vi "sätt_ström_supersub.vi"(5 "Spänningsaggregat":refnum<visa-resource-name>="COM4", 7 "Strömmultimeter":refnum<visa-resource-name>, 8 "error in":errorcluster, 9 "voltage_max":dbl, 10 "current_in":dbl) -> (0 "error out":errorcluster, 2 "current_act":dbl)   [LabVIEW 2024]
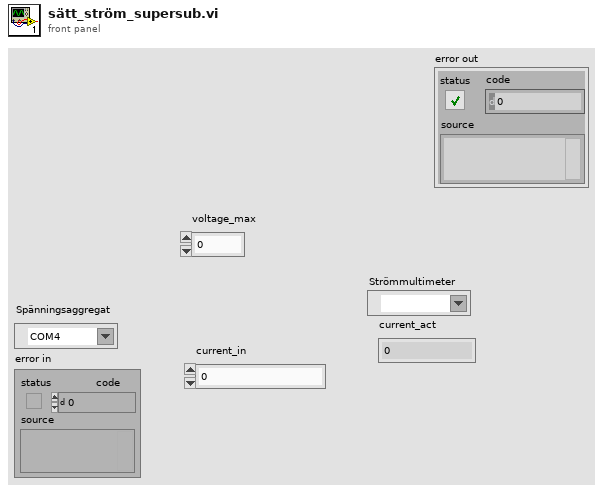
[diagram p1: front panel]
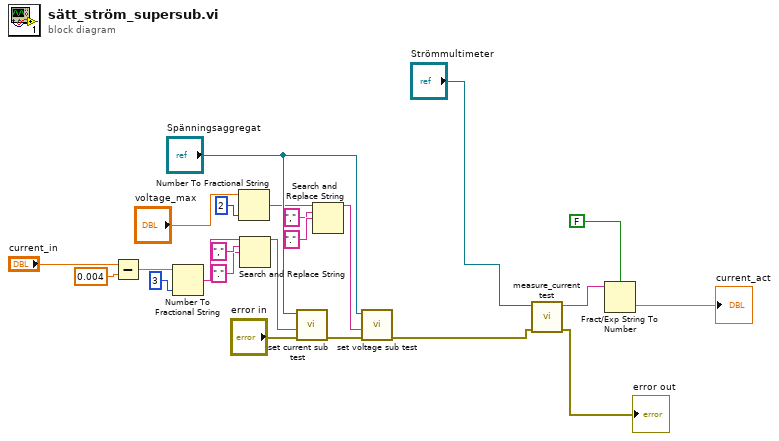
[diagram p0: block diagram]
diagram:
  n1 = Subtract(x="current_in", y=0.004) -> (x-y=w15:dbl)
  n2 = Number To Fractional String(number=w15, precision (6)=i16 3) -> (F-format string=w23:string)  [unwired: 2 in]
  n3 = Number To Fractional String(number="voltage_max", precision (6)=i16 2) -> (F-format string=w10:string)  [unwired: 2 in]
  n4 = Search and Replace String(input string=w23, search string=",", replace string="." ("replace string (\"\")")) -> (result string=w19:string)  [unwired: 5 in, 3 out]
  n5 = call "set current sub test.vi"("error in (no error)"="error in", "result string"=w19, "VISA Refnum in"="Spänningsaggregat") -> ("error out"=w18:errorcluster)  [unwired: 8 in]
  n6 = Search and Replace String(input string=w10, search string=",", replace string="." ("replace string (\"\")")) -> (result string=w7:string)  [unwired: 5 in, 3 out]
  n7 = call "set voltage sub test.vi"("error in (no error)"=w18, "result string"=w7, "VISA Refnum in"="Spänningsaggregat") -> ("error out"=w4:errorcluster)  [unwired: 8 in]
  n8 = call "measure_current test.vi"("error in (no error)"=w4, "VISA Refnum in"="Strömmultimeter") -> ("error out"=→"error out":errorcluster, "read buffer"=w3:string)  [unwired: 8 in]
  n9 = Fract/Exp String To Number(use system decimal point (T)=FALSE, string=w3) -> (number=→"current_act":dbl)  [unwired: 2 in, 1 out]
